vi "test_code_write_to_from_file.vi"() -> ()   [LabVIEW 2013]
panel:
  out "names":string[](array[string])
  out "values":variant
  out "xml string":string
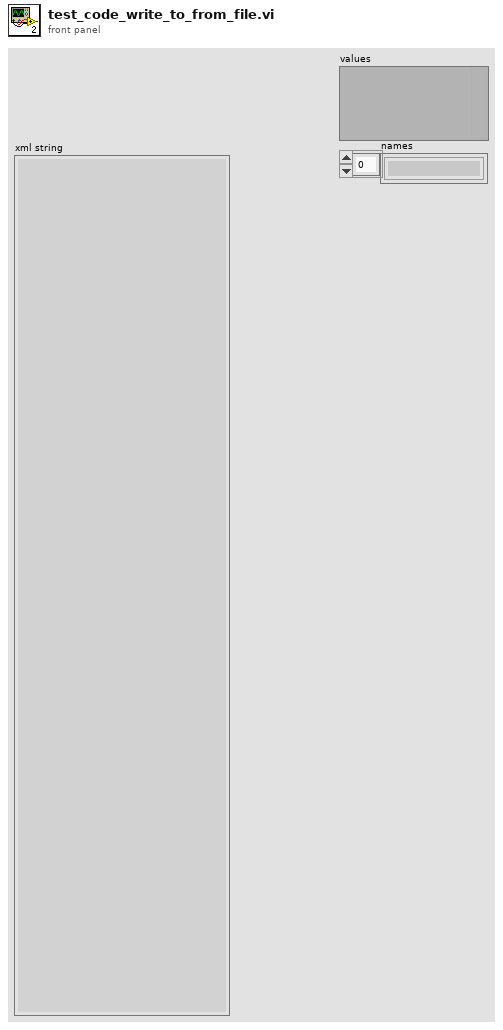
[diagram p1: front panel]
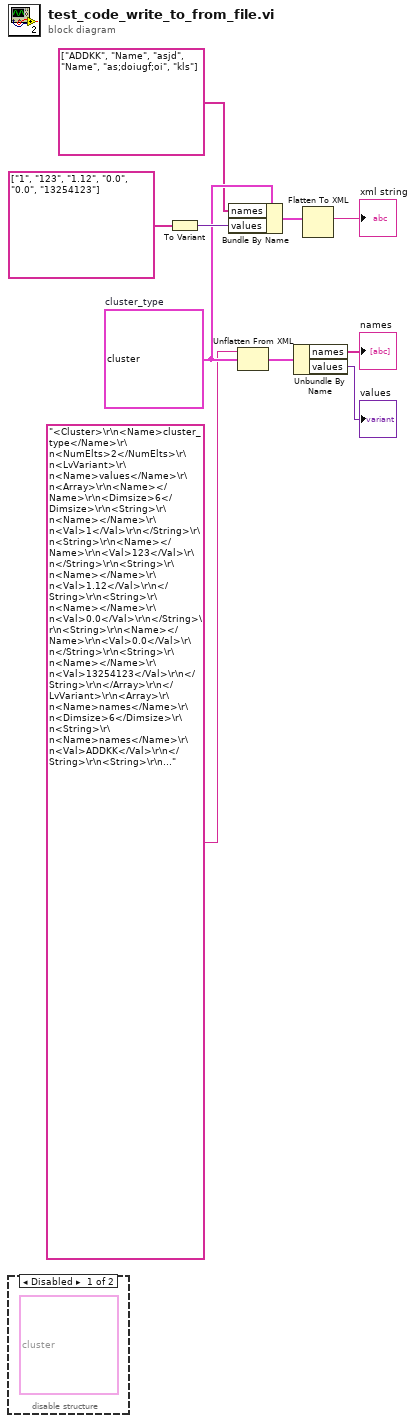
[diagram p0: block diagram]
diagram:
  w6 = cluster{"values":variant, "names":string[]} {"values"=variant, "names"=[]}  # cluster_type
  n1 = disable-structure shown="Disabled" {
    frame Disabled {
      (unwired) cluster{"values":variant, "names":string} {"values"=variant, "names"=""}
    }
    frame Enabled {
    }
  }
  n2 = To Variant(anything=string[] ["1", "123", "1.12", "0.0", "0.0", "13254123"]) -> (Variant=w9:variant)
  n3 = Bundle By Name(cluster=w6, "names"=string[] ["ADDKK", "Name", "asjd", "Name", "as;doiugf;oi", "kls"], "values"=w9) -> (w8:cluster{"values":variant, "names":string[]})
  n4 = Unflatten From XML(xml string="<Cluster>\r\n<Name>cluster_type</Name>\r\n<NumElts>2</NumElts>\r\n<LvVariant>\r\n<Name>values</Name>\r\n<Array>\r\n<Name></Name>\r\n<Dimsize>6</Dimsize>\r\n<String>\r\n<Name></Name>\r\n<Val>1</Val>\r\n</String>\r\n<String>\r\n<Name></Name>\r\n<Val>123</Val>\r\n</String>\r\n<String>\r\n<Name></Name>\r\n<Val>1.12</Val>\r\n</String>\r\n<String>\r\n<Name></Name>\r\n<Val>0.0</Val>\r\n</String>\r\n<String>\r\n<Name></Name>\r\n<Val>0.0</Val>\r\n</String>\r\n<String>\r\n<Name></Name>\r\n<Val>13254123</Val>\r\n</String>\r\n</Array>\r\n</LvVariant>\r\n<Array>\r\n<Name>names</Name>\r\n<Dimsize>6</Dimsize>\r\n<String>\r\n<Name>names</Name>\r\n<Val>ADDKK</Val>\r\n</String>\r\n<String>\r\n<Name>names</Name>\r\n<Val>Name</Val>\r\n</String>\r\n<String>\r\n<Name>names</Name>\r\n<Val>asjd</Val>\r\n</String>\r\n<String>\r\n<Name>names</Name>\r\n<Val>Name</Val>\r\n</String>\r\n<String>\r\n<Name>names</Name>\r\n<Val>as;doiugf;oi</Val>\r\n</String>\r\n<String>\r\n<Name>names</Name>\r\n<Val>kls</Val>\r\n</String>\r\n</Array>\r\n</Cluster>\r\n", type=w6) -> (value=w3:cluster{"values":variant, "names":string[]})  [unwired: 1 in, 1 out]
  n5 = Unbundle By Name(w3) -> ("names"=→"names":string[], "values"=→"values":variant)
  n6 = Flatten To XML(anything=w8) -> (xml string=→"xml string":string)
